vi "syscfg serialize test.vi"() -> ()   [LabVIEW 2014, in "configuration tests.lvlib"]
uses:
  configuration tests.lvlib
  Framework Configuration Classes/system configuration/PL_System Configuration.lvclass
  <vilib>/NI/Configuration Framework/serializable configuration/NISE_CEF_serializable configuration.lvclass/NISE_CEF_serializable configuration.ctl
  Framework Configuration Classes/system configuration/PL_System Configuration.lvclass/PL_System Configuration.ctl
  <vilib>/NI/Configuration Framework/serializable configuration/Read UID.vi
  Framework Configuration Classes/system configuration/Write Configuration Name.vi
  Framework Configuration Classes/system configuration/Write save time.vi
  Framework Configuration Classes/system configuration/Write Saved Version.vi
  Framework Configuration Classes/system configuration/Read Configuration Name.vi
  Framework Configuration Classes/system configuration/Read save time.vi
  Framework Configuration Classes/system configuration/Read Saved Version.vi
  <vilib>/Utility/LVClass/Get LV Class Name.vi
  <vilib>/NI/Configuration Framework/error generator/NISE_error generator.vi
  <vilib>/NI/Configuration Framework/serializable configuration/set alias.vi
  <vilib>/NI/Configuration Framework/serializable configuration/get alias.vi
  <vilib>/NI/Configuration Framework/serializable configuration/NISE_CEF_serializable configuration.lvclass
panel:
  out "verok":bool
  out "timeok":bool
  out "nameok":bool
  out "idok":bool
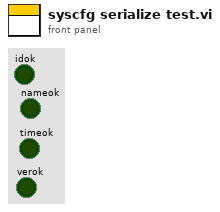
[diagram p1: front panel]
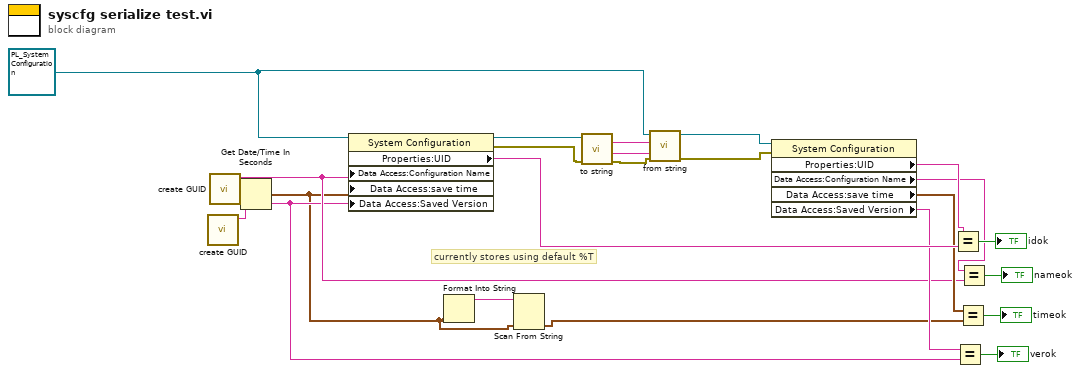
[diagram p0: block diagram]
diagram:
  w20 = refnum<class "PL_System Configuration.lvclass"> refnum ("System Configuration")
  # "currently stores using default %T"
  n1 = call <vilib>:"create GUID.vi"() -> ("uuid"=w6:string)  [unwired: 10 in, 1 out]
  n2 = call <vilib>:"create GUID.vi"() -> ("uuid"=w7:string)  [unwired: 10 in, 1 out]
  n3 = Get Date/Time In Seconds() -> (seconds since 1Jan1904=w2:timestamp)
  n4 = property class="System Configuration"(reference=w20, "Data Access:Configuration Name"=w7, "Data Access:save time"=w2, "Data Access:Saved Version"=w6) -> (reference out=w19:refnum<class "PL_System Configuration.lvclass">, error out=w5:errorcluster, "Properties:UID"=w15:string)  [unwired: 1 in]
  n5 = Format Into String(w2) -> (resulting string=w3:string)  [unwired: 3 in, 1 out]
  n6 = Scan From String(input string=w3, default 1=w2) -> (output 1=w1:timestamp)  [unwired: 3 in, 3 out]
  n7 = call-dynamic "to string.vi"("error in"=w5, "configuration in"=w19) -> ("error out"=w4:errorcluster, "data"=w21:string, "version"=w22:string)  [unwired: 6 in, 1 out]
  n8 = call-dynamic "from string.vi"("error in"=w4, "data"=w21, "version"=w22, "configuration in"=w20) -> ("error out"=w18:errorcluster, "configuration out"=w17:refnum<class "PL_System Configuration.lvclass">)  [unwired: 6 in]
  n9 = property class="System Configuration"(reference=w17, error in=w18) -> ("Properties:UID"=w16:string, "Data Access:Configuration Name"=w8:string, "Data Access:save time"=w9:timestamp, "Data Access:Saved Version"=w10:string)  [unwired: 2 out]
  n10 = Equal?(x=w16, y=w15) -> (x = y?=→"idok":bool)
  n11 = Equal?(x=w10, y=w6) -> (x = y?=→"verok":bool)
  n12 = Equal?(x=w9, y=w1) -> (x = y?=→"timeok":bool)
  n13 = Equal?(x=w8, y=w7) -> (x = y?=→"nameok":bool)
